vi "write basic params.vi"(0 "device_type in":refnum<class "device_type.lvclass">, 1 "buffer size":u32, 2 "Fs  FPGA":dbl, 3 "SPC":dbl, 4 "center frequency (Hz)":dbl, 5 "error in (no error)":errorcluster) -> (14 "device_type out":refnum<class "device_type.lvclass">, 19 "error out":errorcluster)   [LabVIEW 2021, in "device_type.lvclass"]
uses:
  device_type.lvclass
  device_type.lvclass/device_type.ctl
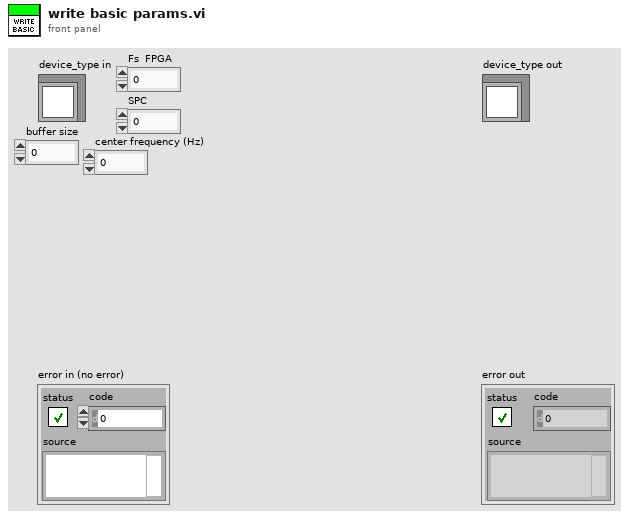
[diagram p1: front panel]
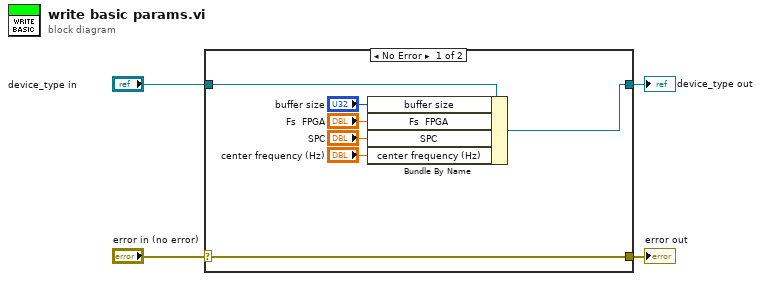
[diagram p0: block diagram]
diagram:
  n1 = case shown="No Error" "error in (no error)" {
    selector: "error in (no error)" -> [w11 w12]
    tunnel: [w11 w12] -> w3
    tunnel: [w9 w13] -> w1
    tunnel: "device_type in" -> [w10 w13]
    frame No Error {
      n2 = Bundle By Name(cluster=w10, "buffer size"="buffer size", "Fs  FPGA"="Fs  FPGA", "SPC"="SPC", "center frequency (Hz)"="center frequency (Hz)") -> (w9:refnum<class "device_type.lvclass">)
    }
    frame Error {
    }
  }
  "error out" <- w3
  "device_type out" <- w1
